vi "ATF - DD Datalog and display modified.vi"() -> ()   [LabVIEW 2022 SP3]
doc: "Datalog and display software modified"
uses:
  Source Code/Control/SeCrTs-Enum.ctl
  Source Code/Globals/SeCrTS-DD globals.vi
panel:
  out "cmd":bool=TRUE
  out "Log Name":string
  out "Storage Connected?":bool
  in  "Storage IP ADDRESS":string="1.1.1.20"
  in  "Exit":bool
  out "Log type":bool
  out "Log Period(Min)":dbl
  in  "Pumb IP ADDRESS":string="169.254.92.110"
  out "Logging?":bool
  out "Pumb Connected?":bool
  out "error Out":errorcluster
  # "VERSION           : V1.2\nRELEASE DATE : 23/09/2024"
  # "DATALOG AND DISPLAY SOFTWARE"
  # "Continuous log"
  # "Periodical log"
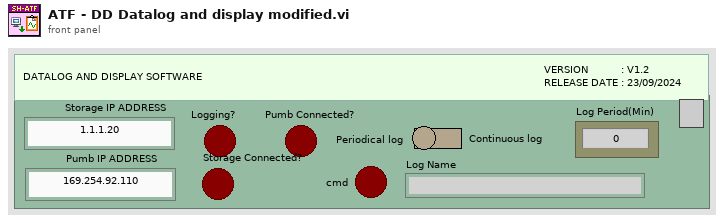
[diagram p1: front panel]
types:
  T1 = typedef "SeCrTs-Enum.ctl" = enum16{"Initialize", "Poll", "Establish ref", "Read", "Close", "Exit"}
  T2 = enum8{"Enabled", "Disabled", "Disabled and Grayed Out"}
  T3 = cluster{"C/NC":bool, "Start/Stop Log":bool[], "Log Name":string, "Config":cluster{"AO config":cluster{"Channel_Name":string, "Channel_Number":string, "Default_Value":dbl, "Units":string}[], "AI config":cluster{"Channel_Name":string, "Channel_Number":string, "Pre_Scale_min":dbl, "Pre_Scale_max":dbl, "Sensor_min":dbl, "Sensor_max":dbl, "Units":string}[], "DI config":cluster{"Channel_Name":string, "Channel_Number":string, "Default_Value":bool, "DI invert?":bool}[], "DO config":cluster{"Channel_Name":string, "Channel_Number":string, "Default_Value":bool, "DO invert?":bool}[], "TC config":cluster{"Channel_Name":string, "Channel_Number":string, "Pre_Scale_min":dbl, "Pre_Scale_max":dbl, "units":i32, " type":i32}[], "ACC config":cluster{"Channel_Name":string, "Channel_Number":string, "Pre_Scale_min":dbl, "Pre_Scale_max":dbl, "Terminal configuration":i32, "Sensitivity":dbl, "Sensitivity units":i32}[], "SG config":cluster{"Channel_Name":string, "Channel_Number":string, "Pre_Scale_min":dbl, "Pre_Scale_max":dbl}[], "Strain Gauge Settings":cluster{"poisson ratio":dbl, "nominal gage resistance":dbl, "gage factor":dbl}, "Bridge Settings":cluster{"voltage excitation value":dbl, "voltage excitation source":i32, "initial bridge voltage":dbl, "lead wire resistance":dbl, "strain configuration":i32}, "Sample Rate":cluster{"AI Sample Rate":dbl[], "AO Sample Rate":dbl[], "DI Sample Rate":dbl[], "TC Sample Rate":dbl[], "DO Sample Rate":dbl[], "SG Sample Rate":dbl[], "ACC Sample Rate":dbl[]}}, "Log min":dbl}
  T4 = cluster{"AO config":cluster{"Channel_Name":string, "Channel_Number":string, "Default_Value":dbl, "Units":string}[], "AI config":cluster{"Channel_Name":string, "Channel_Number":string, "Pre_Scale_min":dbl, "Pre_Scale_max":dbl, "Sensor_min":dbl, "Sensor_max":dbl, "Units":string}[], "DI config":cluster{"Channel_Name":string, "Channel_Number":string, "Default_Value":bool, "DI invert?":bool}[], "DO config":cluster{"Channel_Name":string, "Channel_Number":string, "Default_Value":bool, "DO invert?":bool}[], "TC config":cluster{"Channel_Name":string, "Channel_Number":string, "Pre_Scale_min":dbl, "Pre_Scale_max":dbl, "units":i32, " type":i32}[], "ACC config":cluster{"Channel_Name":string, "Channel_Number":string, "Pre_Scale_min":dbl, "Pre_Scale_max":dbl, "Terminal configuration":i32, "Sensitivity":dbl, "Sensitivity units":i32}[], "SG config":cluster{"Channel_Name":string, "Channel_Number":string, "Pre_Scale_min":dbl, "Pre_Scale_max":dbl}[], "Strain Gauge Settings":cluster{"poisson ratio":dbl, "nominal gage resistance":dbl, "gage factor":dbl}, "Bridge Settings":cluster{"voltage excitation value":dbl, "voltage excitation source":i32, "initial bridge voltage":dbl, "lead wire resistance":dbl, "strain configuration":i32}, "Sample Rate":cluster{"AI Sample Rate":dbl[], "AO Sample Rate":dbl[], "DI Sample Rate":dbl[], "TC Sample Rate":dbl[], "DO Sample Rate":dbl[], "SG Sample Rate":dbl[], "ACC Sample Rate":dbl[]}}
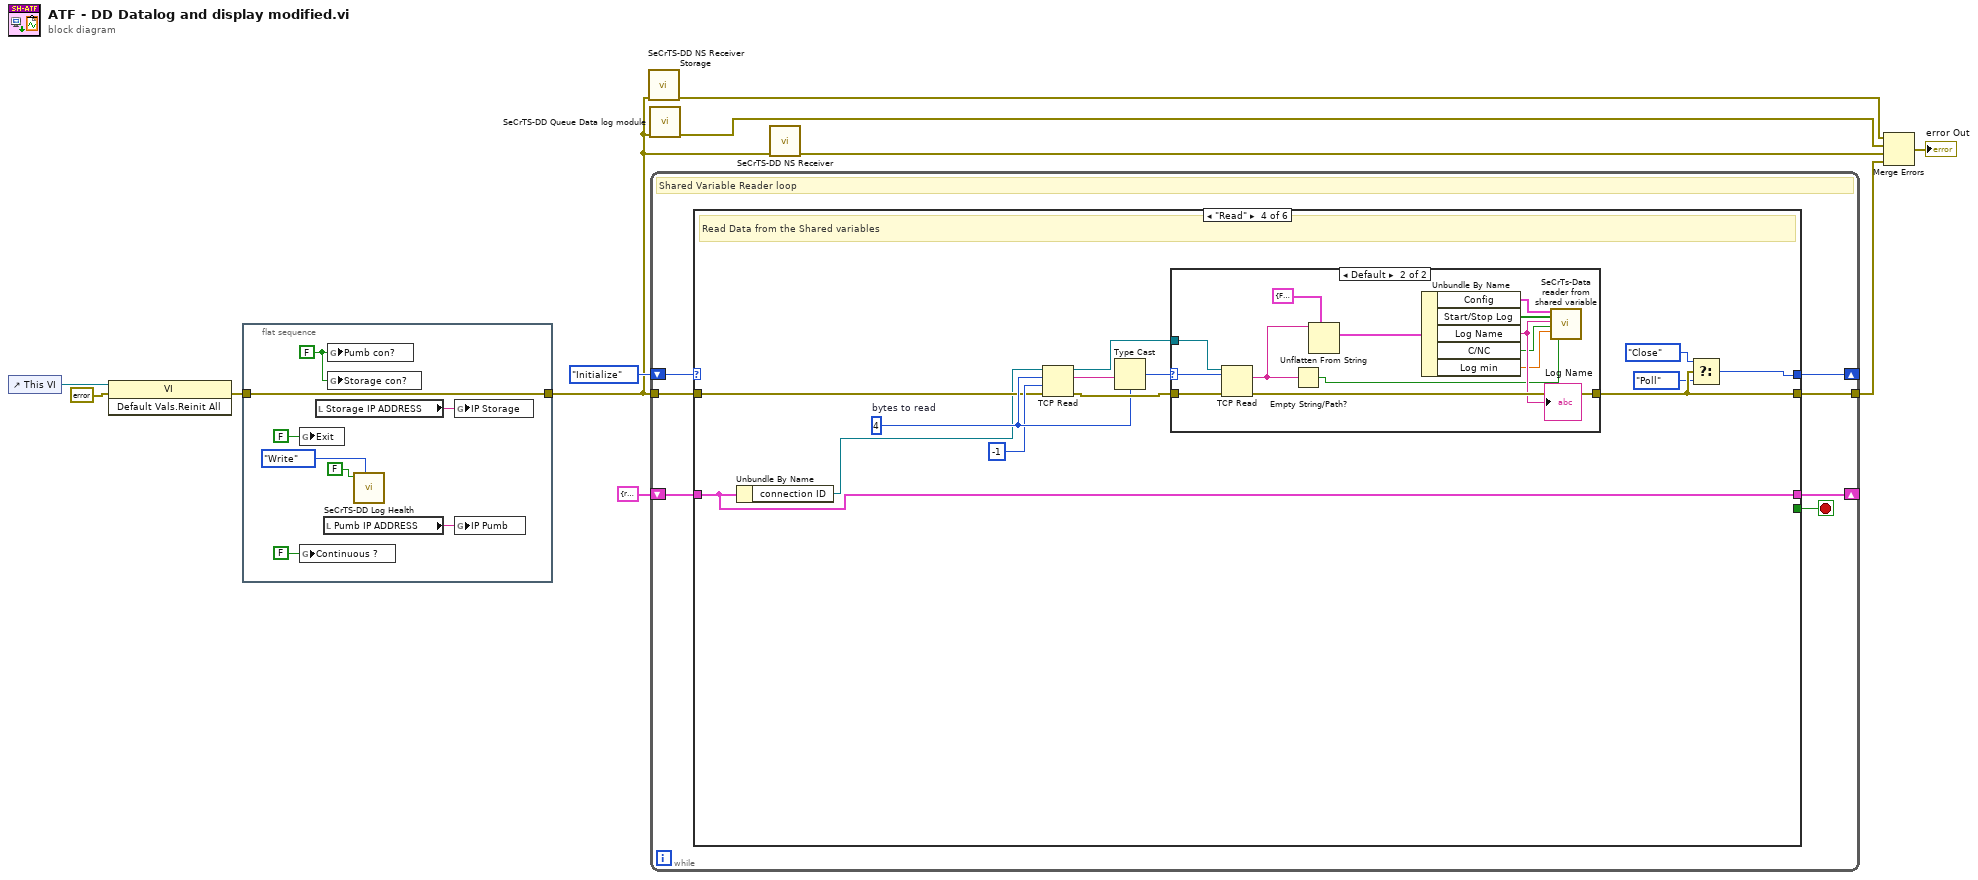
[diagram p0: block diagram]
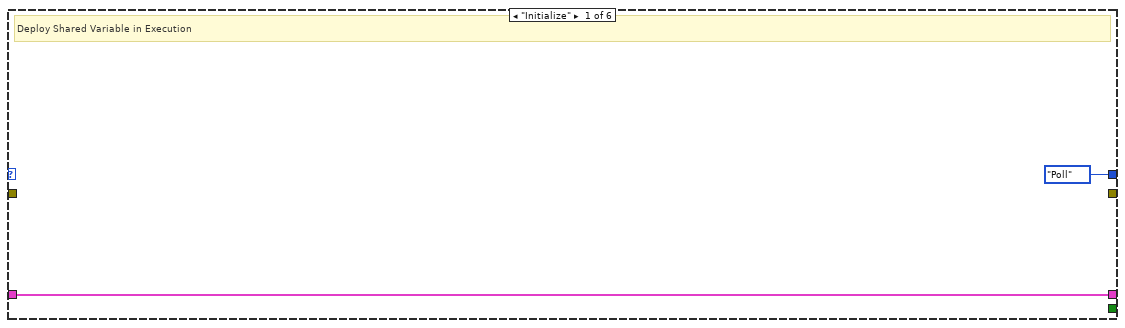
[diagram p2: hidden frame]
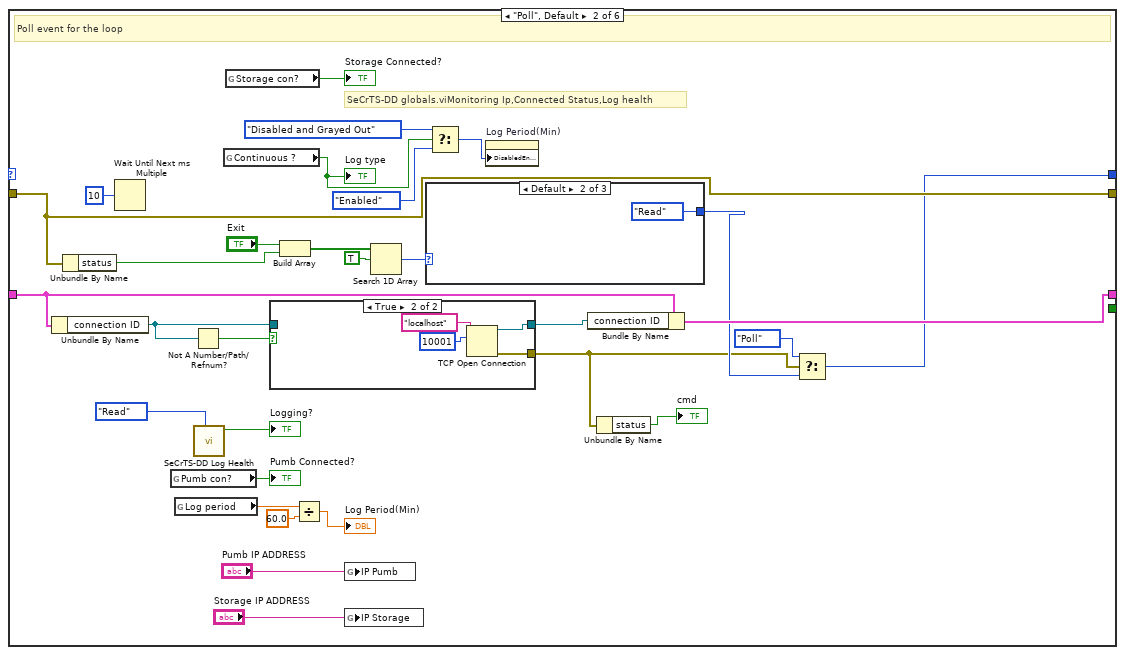
[diagram p3: hidden frame]
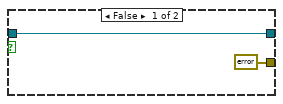
[diagram p4: hidden frame]
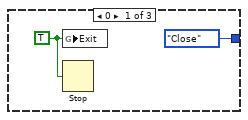
[diagram p5: hidden frame]
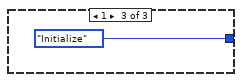
[diagram p6: hidden frame]
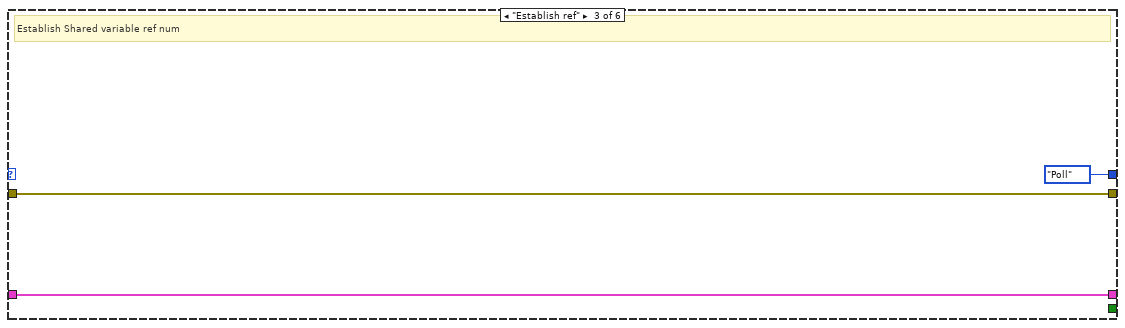
[diagram p7: hidden frame]
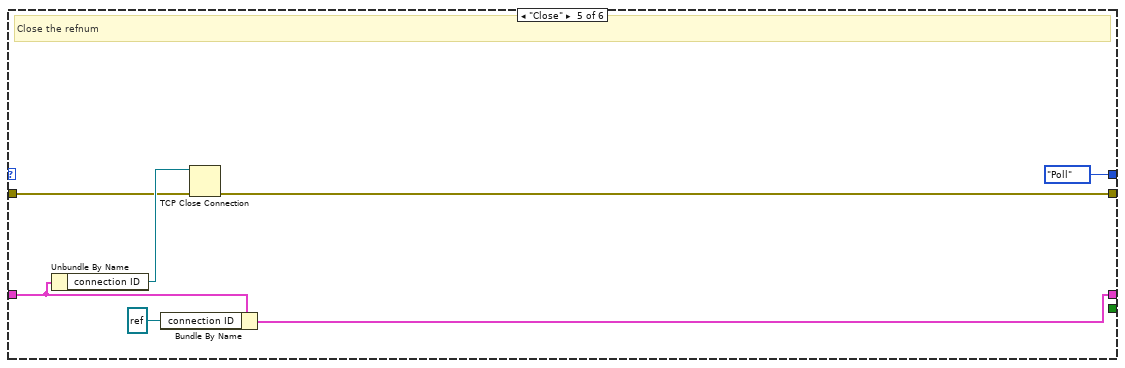
[diagram p9: hidden frame]
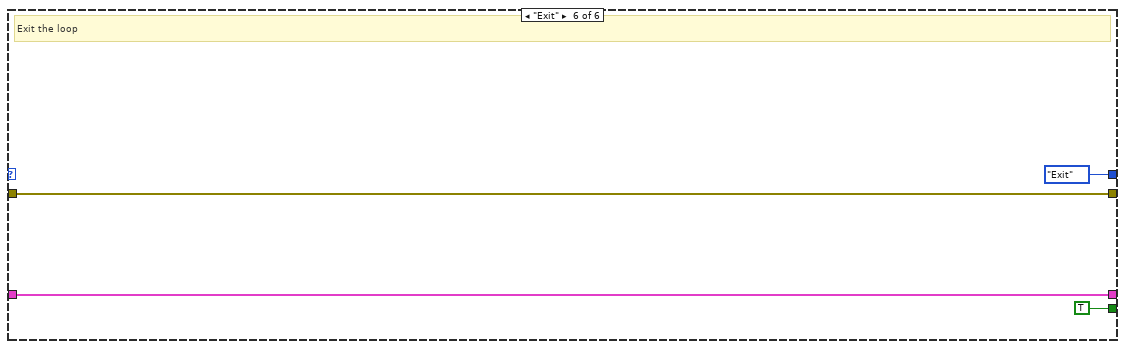
[diagram p10: hidden frame]
diagram:
  n1 = control-ref of="This VI"() -> (w6:refnum<vi>)
  n2 = invoke class="VI" method="Default Vals.Reinit All"(reference=w6, error in=errorcluster {"status"=FALSE, "code"=0, "source"=""}) -> (error out=w4:errorcluster)  [unwired: 1 in, 2 out]
  n3 = flat-sequence {
    tunnel: [w15] -> w3
    tunnel: w4 -> [w15]
    frame #0 {
      w12 = FALSE ("Connect?")
      n4 = global write "SeCrTS-DD globals.vi" "Exit"(FALSE ("EXIT")) -> ()
      n5 = global write "SeCrTS-DD globals.vi" "Continuous ?"(FALSE ("Continuous ?")) -> ()
      n6 = local read "Storage IP ADDRESS"() -> (w13:string)
      n7 = local read "Pumb IP ADDRESS"() -> (w16:string)
      n8 = global write "SeCrTS-DD globals.vi" "Pumb con?"(w12) -> ()
      n9 = global write "SeCrTS-DD globals.vi" "Storage con?"(w12) -> ()
      n10 = call "SeCrTS-DD Log Health.vi"("Enum"=enum16{"Read", "Write"}."Write", "Log health"=FALSE) -> ()  [unwired: 8 in, 2 out]
      n11 = global write "SeCrTS-DD globals.vi" "IP Storage"(w13) -> ()
      n12 = global write "SeCrTS-DD globals.vi" "IP Pumb"(w16) -> ()
    }
  }
  n13 = call "SeCrTS-DD NS Receiver Storage.vi"("error in"=w3) -> ("error out"=w2:errorcluster)  [unwired: 10 in]
  n14 = call "SeCrTS-DD Queue Data log module.vi"("error in"=w3) -> ("error out"=w8:errorcluster)  [unwired: 10 in]
  n15 = while {
    shift-right: [w23] -> _
    shift-left: SeCrTs-Enum."Initialize" -> [w26]
    shift-right: [w21] -> _
    shift-left: cluster{"connection ID":refnum<k5>} {"connection ID"=refnum} -> [w22]
    tunnel: w3 -> [w25]
    tunnel: [w24] -> w10
    stop <- w20 stop-if-true
    # "Shared Variable Reader loop"
    n16 = case shown="\"Read\"" w26 {
      tunnel: w25 -> [_ w39 w70 w79 w103 w107]
      tunnel: [_ w39 w70 w76 w102 w107] -> w24
      tunnel: [SeCrTs-Enum."Poll" w31 SeCrTs-Enum."Poll" w73 SeCrTs-Enum."Poll" SeCrTs-Enum."Exit"] -> w23
      tunnel: w22 -> [w27 w36 w69 w72 w100 w106]
      tunnel: [w27 w38 w69 w72 w101 w106] -> w21
      tunnel: [_ _ _ _ _ TRUE] -> w20
      frame "Initialize" {
        # "Deploy Shared Variable in Execution"
      }
      frame "Poll", Default {
        # "SeCrTS-DD globals.viMonitoring Ip,Connected Status,Log health"
        # "Poll event for the loop"
        n17 = Unbundle By Name(w36) -> ("connection ID"=w34:refnum<k5>)
        n18 = Unbundle By Name(w39) -> ("status"=w58:bool)
        n19 = Wait Until Next ms Multiple(millisecond multiple=u32 10) -> ()  [unwired: 1 out]
        n20 = global read "SeCrTS-DD globals.vi" "Pumb con?"() -> (→"Pumb Connected?":bool)
        n21 = global read "SeCrTS-DD globals.vi" "Log period"() -> (w40:dbl)
        n22 = Not A Number/Path/Refnum?(number/path/refnum=w34) -> (NaN/Path/Refnum?=w35:bool)
        n23 = call "SeCrTS-DD Log Health.vi"("Enum"=enum16{"Read", "Write"}."Read") -> ("Log health R"=→"Logging?":bool)  [unwired: 9 in, 1 out]
        n24 = global read "SeCrTS-DD globals.vi" "Continuous ?"() -> (w45:bool)
        "Log type" <- w45
        n25 = global read "SeCrTS-DD globals.vi" "Storage con?"() -> (→"Storage Connected?":bool)
        n26 = case shown="True" w35 {
          tunnel: [w60 w64] -> w37
          tunnel: w34 -> [w60 _]
          tunnel: [errorcluster {"status"=FALSE, "code"=0, "source"=""} ("error out") w63] -> w30
          frame False {
          }
          frame True {
            n27 = TCP Open Connection(address="localhost", remote port or service name=u16 10001) -> (connection ID=w64:refnum<k5>, error out=w63:errorcluster)  [unwired: 3 in]
          }
        }
        n28 = Build Array("Exit", w58) -> (w56:bool[])
        n29 = Divide(x=w40, y=60.0) -> (x/y=→"Log Period(Min)":dbl)
        n30 = global write "SeCrTS-DD globals.vi" "IP Pumb"("Pumb IP ADDRESS") -> ()
        n31 = global write "SeCrTS-DD globals.vi" "IP Storage"("Storage IP ADDRESS") -> ()
        n32 = Search 1D Array(1D array=w56, element=TRUE) -> (index of element=w57:i32)  [unwired: 1 in]
        n33 = case shown="Default" w57 {
          tunnel: [SeCrTs-Enum."Close" SeCrTs-Enum."Read" SeCrTs-Enum."Initialize"] -> w32
          frame 0 {
            w65 = TRUE ("EXIT")
            n34 = global write "SeCrTS-DD globals.vi" "Exit"(w65) -> ()
            n35 = Stop(stop? (T)=w65) -> ()
          }
          frame Default {
          }
          frame 1 {
          }
        }
        n36 = Select(t=T2."Disabled and Grayed Out" ("Disabled"), s=w45, f=T2."Enabled" ("Disabled")) -> (s? t:f=w46:T2)
        n37 = property on="Log Period(Min)" class="DigNum (strict)"("DisabledEnum"=w46) -> ()  [unwired: 2 in, 2 out]
        n38 = Bundle By Name(cluster=w36, "connection ID"=w37) -> (w38:cluster{"connection ID":refnum<k5>})
        n39 = Unbundle By Name(w30) -> ("status"=→"cmd":bool)
        n40 = Select(t=SeCrTs-Enum."Poll", s=w30, f=w32) -> (s? t:f=w31:T1)
      }
      frame "Establish ref" {
        # "Establish Shared variable ref num"
      }
      frame "Read" {
        w82 = 4  # bytes to read
        # "Read Data from the Shared variables"
        n41 = Unbundle By Name(w72) -> ("connection ID"=w78:refnum<k5>)
        n42 = TCP Read(connection ID=w78, bytes to read=w82, error in (no error)=w79, 9:-1 ("timeout ms (25000)")) -> (connection ID out=w77:refnum<k5>, data out=w84:string, error out=w83:errorcluster)  [unwired: 1 in]
        n43 = Type Cast(type=w82, x=w84) -> (*(type *) &x=w81:i32)
        n44 = case shown="Default" w81 {
          selector: w81 -> [_ w95]
          tunnel: w77 -> [_ w98]
          tunnel: w83 -> [w85 w97]
          tunnel: [w85 w96] -> w76
          frame ..0 {
            # "The server has not written any data"
          }
          frame Default {
            n45 = TCP Read(connection ID=w98, bytes to read=w95, error in (no error)=w97) -> (data out=w87:string, error out=w96:errorcluster)  [unwired: 2 in, 1 out]
            n46 = Empty String/Path?(string/path=w87) -> (empty?=w86:bool)
            n47 = Unflatten From String(type=T3 {"C/NC"=FALSE, "Start/Stop Log"=[], "Log Name"="", "Config"={"AO config"=[], "AI config"=[], "DI config"=[], "DO config"=[], "TC config"=[], "ACC config"=[], "SG config"=[], "Strain Gauge Settings"={"poisson ratio"=0.0, "nominal gage resistance"=0.0, "gage factor"=0.0}, "Bridge Settings"={"voltage excitation value"=0.0, "voltage excitation source"=0, "initial bridge voltage"=0.0, "lead wire resistance"=0.0, "strain configuration"=0}, "Sample Rate"={"AI Sample Rate"=[], "AO Sample Rate"=[], "DI Sample Rate"=[], "TC Sample Rate"=[], "DO Sample Rate"=[], "SG Sample Rate"=[], "ACC Sample Rate"=[]}}, "Log min"=0.0} ("Cluster"), binary string=w87) -> (value=w93:T3)  [unwired: 3 in, 2 out]
            n48 = Unbundle By Name(w93) -> ("Config"=w92:T4, "Start/Stop Log"=w91:bool[], "Log Name"=w90:string, "C/NC"=w89:bool, "Log min"=w88:dbl)
            "Log Name" <- w90
            n49 = call "SeCrTs-Data reader from shared variable.vi"("Config"=w92, "Start/Stop Log"=w91, "Log Name"=w90, "C/NC"=w89, "Log min"=w88, "empty?"=w86) -> ()  [unwired: 13 in, 1 out]
          }
        }
        n50 = Select(t=SeCrTs-Enum."Close", s=w76, f=SeCrTs-Enum."Poll") -> (s? t:f=w73:T1)
      }
      frame "Close" {
        # "Close the refnum"
        n51 = Unbundle By Name(w100) -> ("connection ID"=w104:refnum<k5>)
        n52 = Bundle By Name(cluster=w100, "connection ID"=refnum<k5> refnum) -> (w101:cluster{"connection ID":refnum<k5>})
        n53 = TCP Close Connection(connection ID=w104, error in (no error)=w103) -> (error out=w102:errorcluster)  [unwired: 1 in, 1 out]
      }
      frame "Exit" {
        # "Exit the loop"
      }
    }
  }
  n54 = call "SeCrTS-DD NS Receiver.vi"("error in"=w3) -> ("error out"=w7:errorcluster)  [unwired: 10 in]
  n55 = Merge Errors(w2, w8, w7, w10) -> (→"error Out":errorcluster)
